vi "Helper.vi"() -> ()   [LabVIEW 2015]
uses:
  Application Specific/Actors/Launcher/Actor/Launcher Actor.lvclass
  Application Specific/Actors/Main Controller/Actor/Main Controller Actor.lvclass
panel:
  in  "Run?":bool=TRUE
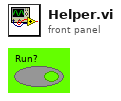
[diagram p1: front panel]
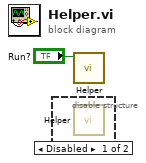
[diagram p0: block diagram]
diagram:
  n1 = disable-structure shown="Disabled" {
    frame Disabled {
      n2 = call "Helper.vi"() -> ()  [unwired: 12 in]
    }
    frame Enabled {
    }
  }
  n3 = call "Helper.vi"("Run?"="Run?") -> ()  [unwired: 11 in]
